vi "Configure Server Group.vi"(8 "error in":errorcluster, 9 "group name":string, 10 "data string":string, 11 "connection info in":T1) -> (0 "error out":errorcluster, 1 "tags exist?":bool)   [LabVIEW 2010, in "NI_CCC.lvlib"]
uses:
  NI_CCC.lvlib
  <vilib>/NI/STM/TCP/TCP Connection Info.ctl
  <vilib>/NI/STM/SubVIs/MetaDataElement.ctl
  Configure Read_Write Message.ctl
  Type_Tag.ctl
  <vilib>/NI/Current Value Table/Type Defs/Data Types.ctl
  <vilib>/NI/Current Value Table/FGVs/Group Memory Methods.ctl
  <vilib>/NI/Current Value Table/FGVs/Tag Memory.vi
  <vilib>/NI/Current Value Table/Form Single Group.vi
  <vilib>/NI/STM/TCP/Write Message (TCP).vi
  <vilib>/NI/Current Value Table/Current Value Table.lvlib
  <vilib>/NI/STM/NI STM.lvlib
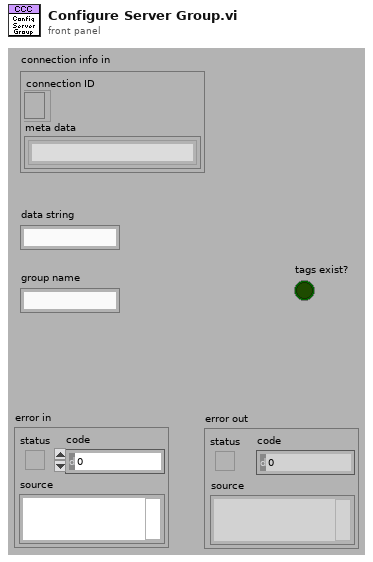
[diagram p1: front panel]
types:
  T1 = typedef "NI STM.lvlib/TCP Connection Info.ctl" = cluster{"connection ID":refnum<k5>, "meta data":T2[]}
  T2 = typedef "NI STM.lvlib/MetaDataElement.ctl" = string
  T3 = typedef "NI_CCC.lvlib/Configure Read_Write Message.ctl" = cluster{"items":T4[]}
  T4 = typedef "NI_CCC.lvlib/Type_Tag.ctl" = cluster{"Data Type":T5, "tag":string}
  T5 = typedef "Current Value Table.lvlib/Data Types.ctl" = enum16{"Double", "Single", "I64", "I32", "I16", "I8", "U64", "U32", "U16", "U8", "String", "Boolean", "Array of U8", "Array of U16", "Array of U32", "Array of U64", "Array of I64", "Array of I32", "Array of I16", "Array of I8", "Array of Double", "Array of Single", "Array of Boolean", "Array of String"}
  T6 = typedef "Current Value Table.lvlib/Group Memory Methods.ctl" = enum16{"Clear", "Read Indices in Group", "List Groups", "List Tags by Type", "List Tags", "Delete Group", "Check Group Existence", "Create Group"}
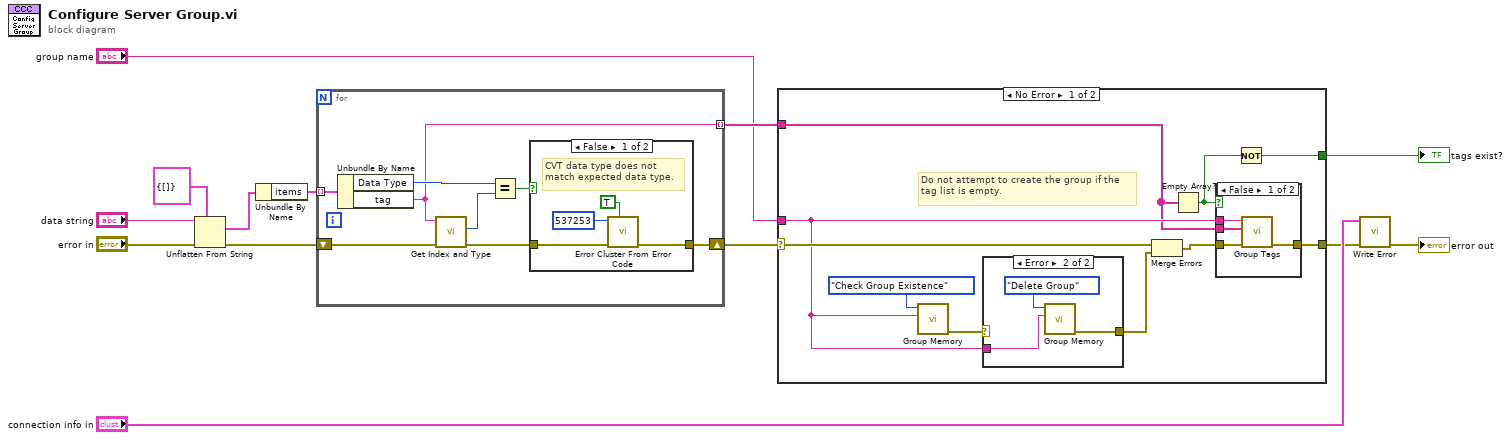
[diagram p0: block diagram]
diagram:
  n1 = Unflatten From String(type=T3 {"items"=[]} ("config write message"), binary string="data string", error in (no error)="error in") -> (value=w10:T3, error out=w11:errorcluster)  [unwired: 3 out]
  n2 = Unbundle By Name(w10) -> ("items"=w2:T4[])
  n3 = for {
    tunnel: w2 -> [w21] mode=indexing
    shift-right: [w18] -> w6
    shift-left: w11 -> [w20]
    tunnel: [w14] -> w4 mode=indexing
    n4 = Unbundle By Name(w21) -> ("Data Type"=w17:T5, "tag"=w14:string)
    n5 = call <vilib>:"Get Index and Type.vi"("error in (no error)"=w20, "Tag"=w14) -> ("error out"=w19:errorcluster, "Type"=w16:T5)  [unwired: 7 in, 1 out]
    n6 = Equal?(x=w17, y=w16) -> (x = y?=w15:bool)
    n7 = case shown="False" w15 {
      tunnel: w19 -> [w24 w26]
      tunnel: [w23 w26] -> w18
      frame False {
        # "CVT data type does not match expected data type."
        n8 = call <vilib>:"Error Cluster From Error Code.vi"("show call chain? (False)"=TRUE, "error in (no error)"=w24, "error code (0)"=537253) -> ("error out"=w23:errorcluster)  [unwired: 6 out]
      }
      frame True {
      }
    }
  }
  n9 = case shown="No Error" w6 {
    selector: w6 -> [w34 w46]
    tunnel: "group name" -> [w30 _]
    tunnel: [w31 w46] -> w5
    tunnel: w4 -> [w29 _]
    tunnel: [w27 _] -> w1
    frame No Error {
      # "Do not attempt to create the group if the tag list is empty."
      n10 = call <vilib>:"Group Memory.vi"("Group"=w30, "Method"=Group_Memory_Methods."Check Group Existence") -> ("error out"=w35:errorcluster)  [unwired: 6 in, 3 out]
      n11 = case shown="Error" w35 {
        selector: w35 -> [w42 _]
        tunnel: w30 -> [_ w44]
        tunnel: [w42 w43] -> w33
        frame No Error {
        }
        frame Error {
          n12 = call <vilib>:"Group Memory.vi"("Group"=w44, "Method"=Group_Memory_Methods."Delete Group") -> ("error out"=w43:errorcluster)  [unwired: 6 in, 3 out]
        }
      }
      n13 = Merge Errors(w34, w33) -> (w32:errorcluster)
      n14 = Empty Array?(array=w29) -> (empty?=w28:bool)
      n15 = case shown="False" w28 {
        tunnel: w32 -> [w40 w41]
        tunnel: [w39 w41] -> w31
        tunnel: w30 -> [w38 _]
        tunnel: w29 -> [w37 _]
        frame False {
          n16 = call <vilib>:"Group Tags.vi"("error in (no error)"=w40, "Tag Names"=w37, "Group"=w38) -> ("error out"=w39:errorcluster)  [unwired: 8 in]
        }
        frame True {
        }
      }
      n17 = Not(x=w28) -> (.not. x?=w27:bool)
    }
    frame Error {
    }
  }
  "tags exist?" <- w1
  n18 = call "Write Error.vi"("error in"=w5, "connection info in"="connection info in") -> ("error out"=→"error out":errorcluster)  [unwired: 9 out]
